vi "Calculator Brainstorming.vi"() -> ()   [LabVIEW 2017]
panel:
  in  "Cancel Button":bool
  in  "stop":bool
  in  "1":bool
  in  "5":bool
  in  "4":bool
  in  "3":bool
  in  "2":bool
  out "Display":dbl
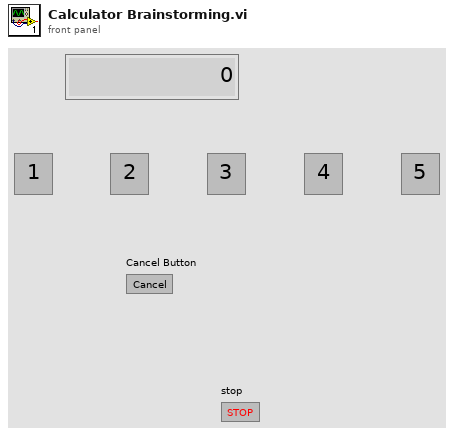
[diagram p1: front panel]
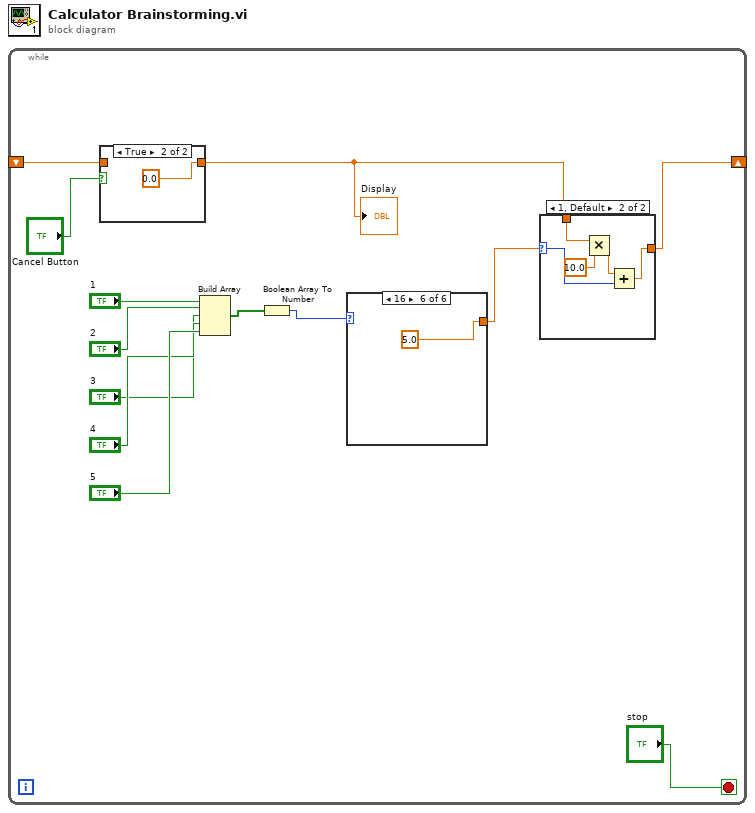
[diagram p0: block diagram]
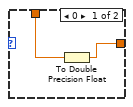
[diagram p3: hidden frame]
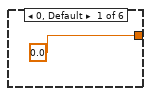
[diagram p4: hidden frame]
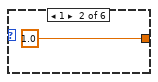
[diagram p5: hidden frame]
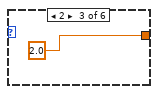
[diagram p6: hidden frame]
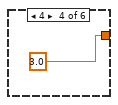
[diagram p7: hidden frame]
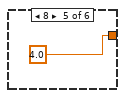
[diagram p8: hidden frame]
diagram:
  n1 = while {
    shift-right: [w5] -> _
    shift-left: _ -> [w2]
    stop <- "stop" stop-if-true
    n2 = case shown="True" "Cancel Button" {
      tunnel: [w14 0.0] -> w3
      tunnel: w2 -> [w14 _]
      frame False {
      }
      frame True {
      }
    }
    "Display" <- w3
    n3 = Build Array("1", "2", "3", "4", "5") -> (w12:bool[])
    n4 = Boolean Array To Number(Boolean array=w12) -> (number=w13:u32)
    n5 = case shown="16" w13 {
      tunnel: [0.0 1.0 2.0 3.0 4.0 5.0] -> w6
      frame 0, Default {
      }
      frame 1 {
      }
      frame 2 {
      }
      frame 4 {
      }
      frame 8 {
      }
      frame 16 {
      }
    }
    n6 = case shown="1, Default" w6 {
      selector: w6 -> [_ w21]
      tunnel: [w16 w18] -> w5
      tunnel: w3 -> [w17 w19]
      frame 0 {
        n7 = To Double Precision Float(number=w17) -> (double precision float=w16:dbl)
      }
      frame 1, Default {
        n8 = Multiply(x=w19, y=10.0) -> (x*y=w22:dbl)
        n9 = Add(x=w22, y=w21) -> (x+y=w18:dbl)
      }
    }
  }
